vi "PathPlanner_Util_TrajStatesToPathPlannerStates.vi"(11 "TrajStates":T1[](array[typedef]) {"POSE"."ROTATION"."SIN" format="%13.4f"; "POSE"."ROTATION"."COS" format="%13.4f"; "POSE"."ROTATION"."VALUE" format="%13.4f"; "POSE"."TRANSLATION"."Y" format="%14.3f"; "POSE"."TRANSLATION"."X" format="%14.3f"}) -> (3 "PathPlannerStates":T5[](array[typedef]) {"HolonomicRotation"."SIN" format="%13.4f"; "HolonomicRotation"."COS" format="%13.4f"; "HolonomicRotation"."VALUE" format="%13.4f"; "AngularVelocity"."SIN" format="%13.4f"; "AngularVelocity"."COS" format="%13.4f"; "AngularVelocity"."VALUE" format="%13.4f"; "TrajectoryState"."POSE"."ROTATION"."SIN" format="%13.4f"; "TrajectoryState"."POSE"."ROTATION"."COS" format="%13.4f"; "TrajectoryState"."POSE"."ROTATION"."VALUE" format="%13.4f"; "TrajectoryState"."POSE"."TRANSLATION"."Y" format="%14.3f"; "TrajectoryState"."POSE"."TRANSLATION"."X" format="%14.3f"; "AngularAcceleration"."SIN" format="%13.4f"; "AngularAcceleration"."COS" format="%13.4f"; "AngularAcceleration"."VALUE" format="%13.4f"})   [LabVIEW 2019]
uses:
  <vilib>/Rock Robotics/WPI/ThirdParty/MJansen/PathPlanner/PathPlannerState.ctl
  <vilib>/Rock Robotics/WPI/ThirdParty/JAS_Junk/TrajLib/ROTATION2D.ctl
  <vilib>/Rock Robotics/WPI/ThirdParty/JAS_Junk/TrajLib/TRAJ_STATE.ctl
  <vilib>/Rock Robotics/WPI/ThirdParty/JAS_Junk/TrajLib/POSE2D.ctl
  <vilib>/Rock Robotics/WPI/ThirdParty/JAS_Junk/TrajLib/TRANSLATION2D.ctl
  <vilib>/Rock Robotics/WPI/ThirdParty/JAS_Junk/TrajLib/Rotation2d_UnaryMinus.vi
  <vilib>/Rock Robotics/WPI/ThirdParty/JAS_Junk/TrajLib/Rotation2d_RotateBy.vi
  <vilib>/Rock Robotics/WPI/ThirdParty/JAS_Junk/TrajLib/Util_CalcDist.vi
  <vilib>/Rock Robotics/WPI/ThirdParty/JAS_Junk/TrajLib/Rotation2d_CreateAngle.vi
  <vilib>/Rock Robotics/WPI/ThirdParty/JAS_Junk/TrajLib/Rotation2d_CreateXY.vi
  <vilib>/Rock Robotics/WPI/ThirdParty/JAS_Junk/TrajLib/Trajectory_Library.lvlib
  <vilib>/Rock Robotics/WPI/ThirdParty/MJansen/PathPlanner/PathPlanner.lvlib
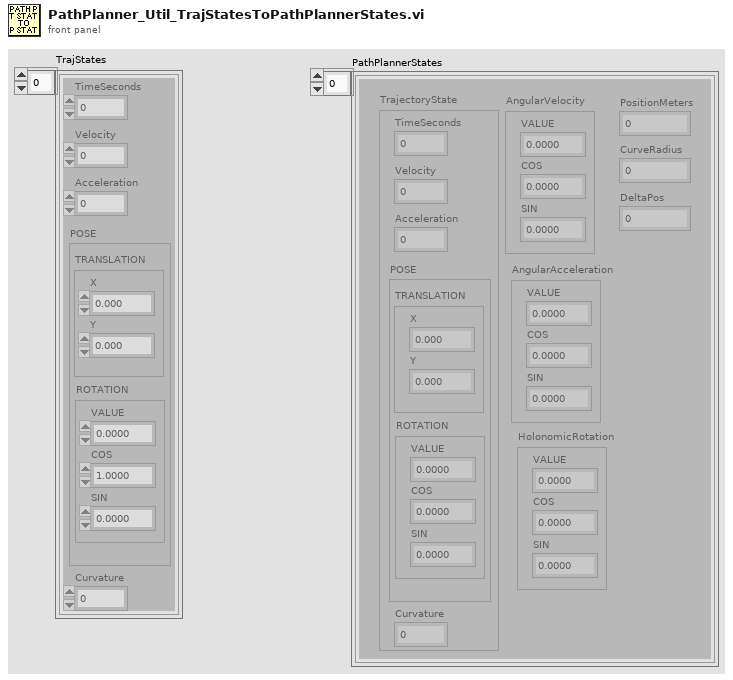
[diagram p1: front panel]
types:
  T1 = typedef "Trajectory_Library.lvlib/TRAJ_STATE.ctl" = cluster{"TimeSeconds":dbl, "Velocity":dbl, "Acceleration":dbl, "POSE":T2, "Curvature":dbl}
  T2 = typedef "Trajectory_Library.lvlib/POSE2D.ctl" = cluster{"TRANSLATION":T3, "ROTATION":T4}
  T3 = typedef "Trajectory_Library.lvlib/TRANSLATION2D.ctl" = cluster{"X":dbl, "Y":dbl}
  T4 = typedef "Trajectory_Library.lvlib/ROTATION2D.ctl" = cluster{"VALUE":dbl, "COS":dbl, "SIN":dbl}
  T5 = typedef "PathPlanner.lvlib/PathPlannerState.ctl" = cluster{"AngularAcceleration":T4, "PositionMeters":dbl, "TrajectoryState":T1, "AngularVelocity":T4, "HolonomicRotation":T4, "CurveRadius":dbl, "DeltaPos":dbl}
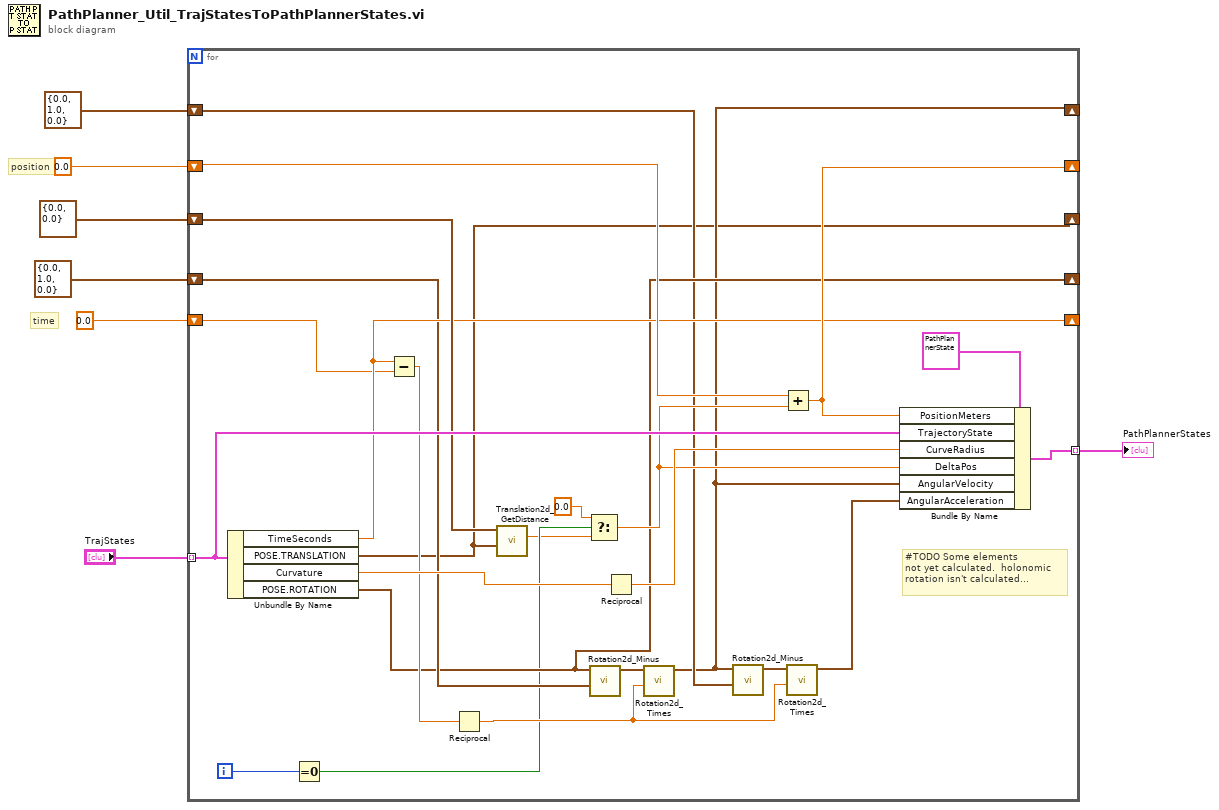
[diagram p0: block diagram]
diagram:
  # "time"
  # "position"
  n1 = for {
    tunnel: "TrajStates" -> [w30] mode=indexing
    tunnel: [w31] -> w7 mode=indexing
    shift-right: [w10] -> _
    shift-left: T3 {"X"=0.0, "Y"=0.0} ("TRANSLATION") -> [w27]
    shift-right: [w23] -> _
    shift-left: 0.0 -> [w24]
    shift-right: [w15] -> _
    shift-left: T4 {"VALUE"=0.0, "COS"=1.0, "SIN"=0.0} ("ROTATION") -> [w16]
    shift-right: [w22] -> _
    shift-left: 0.0 -> [w21]
    shift-right: [w13] -> _
    shift-left: T4 {"VALUE"=0.0, "COS"=1.0, "SIN"=0.0} ("ROTATION") -> [w14]
    i -> [w26]
    # "#TODO Some elements\nnot yet calculated.  holonomic\nrotation isn't calculated..."
    n2 = Unbundle By Name(w30) -> ("TimeSeconds"=w22:dbl, "POSE.TRANSLATION"=w10:T3, "Curvature"=w29:dbl, "POSE.ROTATION"=w15:T4)
    n3 = Equal To 0?(x=w26) -> (x = 0?=w11:bool)
    n4 = Subtract(x=w22, y=w21) -> (x-y=w18:dbl)
    n5 = Reciprocal(x=w18) -> (1/x=w17:dbl)
    n6 = call <vilib>:"Translation2d_GetDistance.vi"("other Translation"=w10, "In Translation"=w27) -> ("Distance"=w9:dbl)  [unwired: 9 in]
    n7 = Select(t=0.0, s=w11, f=w9) -> (s? t:f=w25:dbl)
    n8 = call <vilib>:"Rotation2d_Minus.vi"("other ROTATION"=w16, "in ROTATION"=w15) -> ("out ROTATION"=w20:T4)  [unwired: 9 in]
    n9 = Reciprocal(x=w29) -> (1/x=w28:dbl)
    n10 = call <vilib>:"Rotation2d_Times.vi"("Scalar"=w17, "in ROTATION"=w20) -> ("out ROTATION"=w13:T4)  [unwired: 9 in]
    n11 = call <vilib>:"Rotation2d_Minus.vi"("other ROTATION"=w14, "in ROTATION"=w13) -> ("out ROTATION"=w19:T4)  [unwired: 9 in]
    n12 = Add(x=w24, y=w25) -> (x+y=w23:dbl)
    n13 = call <vilib>:"Rotation2d_Times.vi"("Scalar"=w17, "in ROTATION"=w19) -> ("out ROTATION"=w12:T4)  [unwired: 9 in]
    n14 = Bundle By Name(cluster=T5 {"AngularAcceleration"={"VALUE"=0.0, "COS"=1.0, "SIN"=0.0}, "PositionMeters"=0.0, "TrajectoryState"={"TimeSeconds"=0.0, "Velocity"=0.0, "Acceleration"=0.0, "POSE"={"TRANSLATION"={"X"=0.0, "Y"=0.0}, "ROTATION"={"VALUE"=0.0, "COS"=1.0, "SIN"=0.0}}, "Curvature"=0.0}, "AngularVelocity"={"VALUE"=0.0, "COS"=1.0, "SIN"=0.0}, "HolonomicRotation"={"VALUE"=0.0, "COS"=1.0, "SIN"=0.0}, "CurveRadius"=0.0, "DeltaPos"=0.0} ("PathPlannerState"), "PositionMeters"=w23, "TrajectoryState"=w30, "CurveRadius"=w28, "DeltaPos"=w25, "AngularVelocity"=w13, "AngularAcceleration"=w12) -> (w31:T5)
  }
  "PathPlannerStates" <- w7
